vi "BME_Set_OutputLevel.vi"(7 "DG_Number":i32, 8 "error in (no error)":errorcluster, 10 "PulseWidth in Clockticks":u32, 11 "SignalTypel":T1 items=["TTL"=1, "ECL"=2, "NIM"=3]) -> (0 "error out":errorcluster, 3 "return value":i32)   [LabVIEW 2009]
uses:
  SignalType.ctl
  BME Beispiele/BME DLL/DelayGenerator.dll
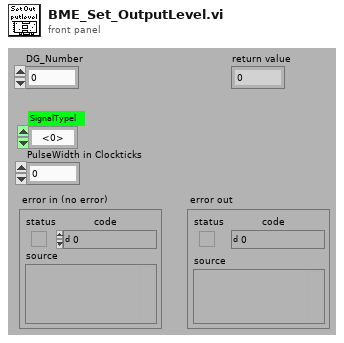
[diagram p1: front panel]
types:
  T1 = typedef "SignalType.ctl" = u32
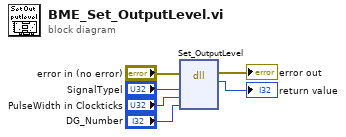
[diagram p0: block diagram]
diagram:
  n1 = dll-call lib="C:/Dokumente und Einstellungen/A2.5/Desktop/BME Beispiele/BME DLL/DelayGenerator.dll" fn="Set_OutputLevel" label="Set Output Level"(error in="error in (no error)", "output  level"="SignalTypel", "pulse width"="PulseWidth in Clockticks", "dg_number"="DG_Number") -> (error out=→"error out":errorcluster, "return type"=→"return value":i32)  [unwired: 5 in, 1 out]
